vi "Unflatten.vi"(8 "error in (no error)":errorcluster, 11 "Pulse Gen Scan in":refnum<class "Pulse Gen Scan.lvclass">) -> (0 "error out":errorcluster, 3 "Pulse Gen Scan out":refnum<class "Pulse Gen Scan.lvclass">)   [LabVIEW 2009, in "Pulse Gen Scan.lvclass"]
uses:
  Pulse Gen Scan.lvclass
  Scanner/Scanner.lvclass
  Global/File Locations.vi
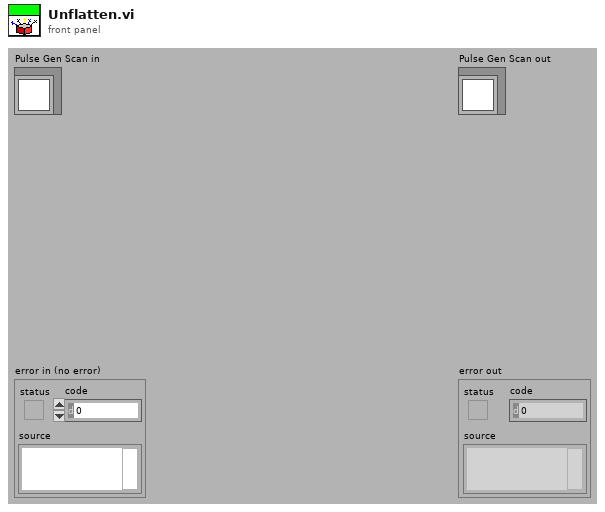
[diagram p1: front panel]
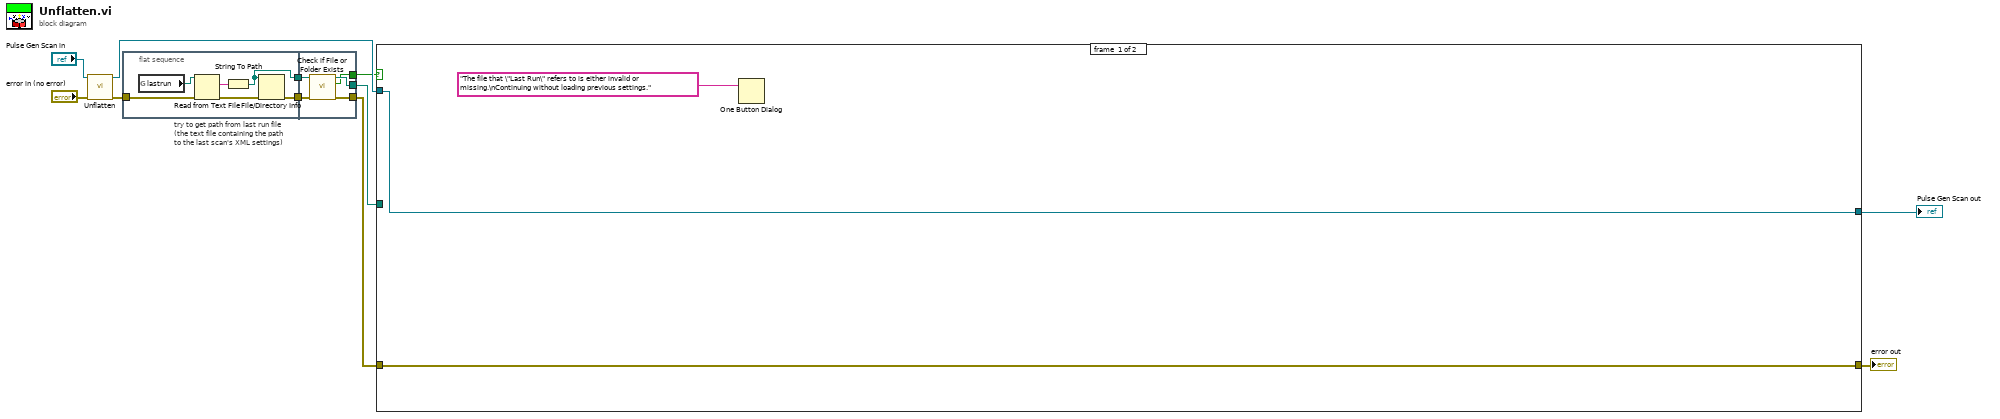
[diagram p0: block diagram]
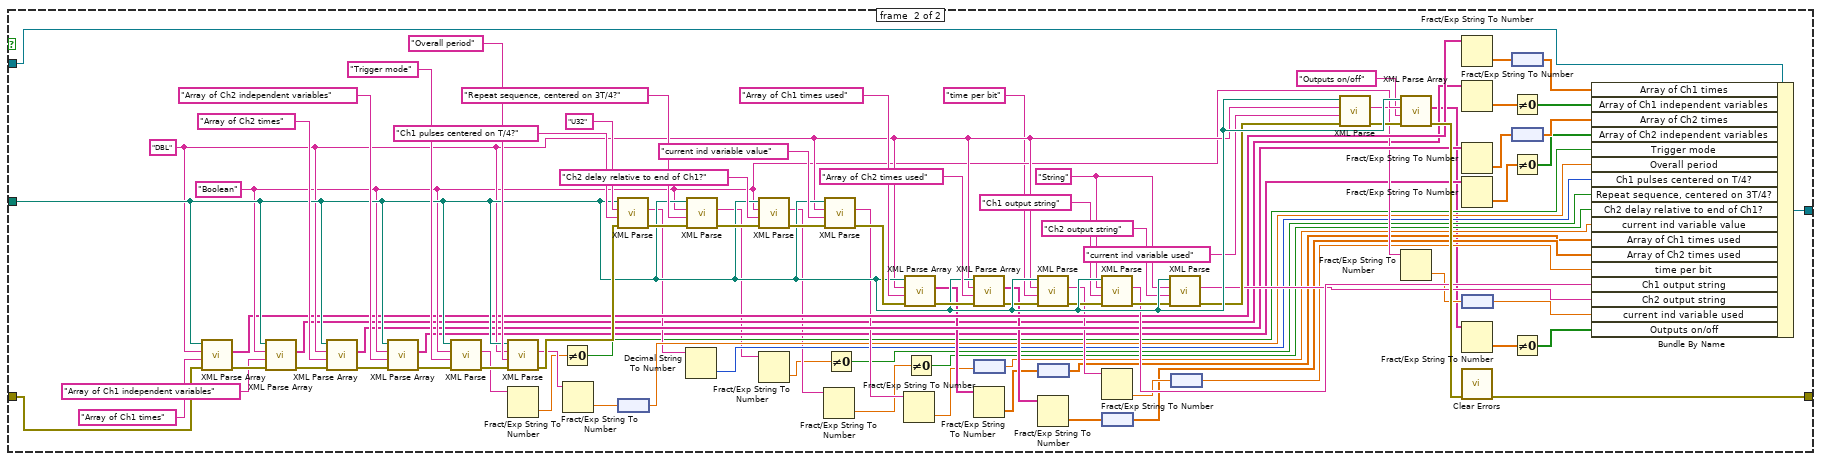
[diagram p2: hidden frame]
diagram:
  n1 = call-parent "Unflatten.vi"("error in (no error)"="error in (no error)", "Scanner in"="Pulse Gen Scan in") -> ("error out"=w7:errorcluster, "Scanner out"=w11:refnum<class "Pulse Gen Scan.lvclass">)  [unwired: 8 in]
  n2 = flat-sequence "try to get path from last run file\n(the text file containing the path\nto the last scan's XML settings)" {
    tunnel: w7 -> [w13]
    tunnel: [w17] -> w3
    tunnel: [w12] -> w2
    tunnel: [w20] -> w6
    tunnel: [w19] -> w5
    tunnel: w3 -> [w22]
    tunnel: w2 -> [w21]
    tunnel: [w18] -> w1
    frame #0 {
      n3 = global read "File Locations.vi" "lastrun"() -> (w15:path)
      n4 = Read from Text File(file (use dialog)=w15, error in=w13) -> (text=w16:string, error out=w14:errorcluster)  [unwired: 4 out]
      n5 = String To Path(string=w16) -> (path=w17:path)
      n6 = File/Directory Info(path=w17, error in=w14) -> (error out=w12:errorcluster)  [unwired: 6 out]
    }
    frame #1 {
      n7 = call <vilib>:"Check if File or Folder Exists.vi"("error in (no error)"=w21, "path"=w22) -> ("error out"=w20:errorcluster, "file or folder exists?"=w18:bool, "dup path"=w19:path)  [unwired: 7 in]
    }
  }
  n8 = case shown="True" w1 {
    tunnel: w11 -> [w24 w114]
    tunnel: [w24 w113] -> w8
    tunnel: w6 -> [w23 w112]
    tunnel: w5 -> [_ w87]
    tunnel: [w23 w26] -> w4
    frame #0 {
      n9 = One Button Dialog(message="The file that \"Last Run\" refers to is either invalid or missing.\nContinuing without loading previous settings.") -> ()  [unwired: 1 in, 1 out]
    }
    frame #1 {
      w86 = "String"
      w84 = "Boolean"
      w85 = "DBL"
      n10 = call "XML Parse Array.vi"("error in (no error)"=w112, "Name String"="Array of Ch1 times", "Type String"=w85, "Path"=w87) -> ("error out"=w111:errorcluster, "Array"=w70:string[])  [unwired: 5 in]
      n11 = call "XML Parse Array.vi"("error in (no error)"=w111, "Name String"="Array of Ch1 independent variables", "Type String"=w84, "Path"=w87) -> ("error out"=w110:errorcluster, "Array"=w44:string[])  [unwired: 5 in]
      n12 = call "XML Parse Array.vi"("error in (no error)"=w110, "Name String"="Array of Ch2 times", "Type String"=w85, "Path"=w87) -> ("error out"=w109:errorcluster, "Array"=w69:string[])  [unwired: 5 in]
      n13 = call "XML Parse Array.vi"("error in (no error)"=w109, "Name String"="Array of Ch2 independent variables", "Type String"=w84, "Path"=w87) -> ("error out"=w104:errorcluster, "Array"=w41:string[])  [unwired: 5 in]
      n14 = call "XML Parse.vi"("error in (no error)"=w104, "Name String"="Trigger mode", "Type String"=w84, "Path"=w87) -> ("error out"=w103:errorcluster, "String Out"=w36:string)  [unwired: 6 in]
      n15 = call "XML Parse.vi"("error in (no error)"=w103, "Name String"="Overall period", "Type String"=w85, "Path"=w87) -> ("error out"=w102:errorcluster, "String Out"=w68:string)  [unwired: 6 in]
      n16 = Fract/Exp String To Number(string=w36) -> (number=w37:dbl)  [unwired: 3 in, 1 out]
      n17 = Not Equal To 0?(x=w37) -> (x != 0?=w38:bool)
      n18 = Fract/Exp String To Number(string=w68) -> (number=w51:dbl)  [unwired: 3 in, 1 out]
      n19 = call "XML Parse.vi"("error in (no error)"=w102, "Name String"="Ch1 pulses centered on T/4?", "Type String"="U32", "Path"=w87) -> ("error out"=w101:errorcluster, "String Out"=w46:string)  [unwired: 6 in]
      n20 = node(w51) -> (w52:dbl[unit])
      n21 = Decimal String To Number(string=w46) -> (number=w45:i32)  [unwired: 2 in, 1 out]
      n22 = call "XML Parse.vi"("error in (no error)"=w101, "Name String"="Repeat sequence, centered on 3T/4?", "Type String"=w84, "Path"=w87) -> ("error out"=w100:errorcluster, "String Out"=w35:string)  [unwired: 6 in]
      n23 = call "XML Parse.vi"("error in (no error)"=w100, "Name String"="Ch2 delay relative to end of Ch1?", "Type String"=w84, "Path"=w87) -> ("error out"=w99:errorcluster, "String Out"=w34:string)  [unwired: 6 in]
      n24 = Fract/Exp String To Number(string=w35) -> (number=w33:dbl)  [unwired: 3 in, 1 out]
      n25 = Fract/Exp String To Number(string=w34) -> (number=w30:dbl)  [unwired: 3 in, 1 out]
      n26 = call "XML Parse.vi"("error in (no error)"=w99, "Name String"="current ind variable value", "Type String"=w85, "Path"=w87) -> ("error out"=w89:errorcluster, "String Out"=w67:string)  [unwired: 6 in]
      n27 = Not Equal To 0?(x=w33) -> (x != 0?=w32:bool)
      n28 = Fract/Exp String To Number(string=w67) -> (number=w53:dbl)  [unwired: 3 in, 1 out]
      n29 = call "XML Parse Array.vi"("error in (no error)"=w89, "Name String"="Array of Ch1 times used", "Type String"=w85, "Path"=w87) -> ("error out"=w88:errorcluster, "Array"=w66:string[])  [unwired: 5 in]
      n30 = Not Equal To 0?(x=w30) -> (x != 0?=w31:bool)
      n31 = call "XML Parse Array.vi"("error in (no error)"=w88, "Name String"="Array of Ch2 times used", "Type String"=w85, "Path"=w87) -> ("error out"=w83:errorcluster, "Array"=w65:string[])  [unwired: 5 in]
      n32 = node(w53) -> (w54:dbl[unit])
      n33 = Fract/Exp String To Number(string=w66) -> (number=w56:dbl[])  [unwired: 3 in, 1 out]
      n34 = call "XML Parse.vi"("error in (no error)"=w83, "Name String"="time per bit", "Type String"=w85, "Path"=w87) -> ("error out"=w82:errorcluster, "String Out"=w64:string)  [unwired: 6 in]
      n35 = node(w56) -> (w55:dbl[unit][])
      n36 = Fract/Exp String To Number(string=w65) -> (number=w57:dbl[])  [unwired: 3 in, 1 out]
      n37 = call "XML Parse.vi"("error in (no error)"=w82, "Name String"="Ch1 output string", "Type String"=w86, "Path"=w87) -> ("error out"=w81:errorcluster, "String Out"=w72:string)  [unwired: 6 in]
      n38 = Fract/Exp String To Number(string=w64) -> (number=w60:dbl)  [unwired: 3 in, 1 out]
      n39 = node(w57) -> (w58:dbl[unit][])
      n40 = call "XML Parse.vi"("error in (no error)"=w81, "Name String"="Ch2 output string", "Type String"=w86, "Path"=w87) -> ("error out"=w80:errorcluster, "String Out"=w71:string)  [unwired: 6 in]
      n41 = node(w60) -> (w59:dbl[unit])
      n42 = call "XML Parse.vi"("error in (no error)"=w80, "Name String"="current ind variable used", "Type String"=w85, "Path"=w87) -> ("error out"=w79:errorcluster, "String Out"=w63:string)  [unwired: 6 in]
      n43 = call "XML Parse Array.vi"("error in (no error)"=w79, "Name String"="Outputs on/off", "Type String"=w84, "Path"=w87) -> ("error out"=w78:errorcluster, "Array"=w27:string[])  [unwired: 5 in]
      n44 = Fract/Exp String To Number(string=w63) -> (number=w61:dbl)  [unwired: 3 in, 1 out]
      n45 = Fract/Exp String To Number(string=w70) -> (number=w47:dbl[])  [unwired: 3 in, 1 out]
      n46 = Fract/Exp String To Number(string=w44) -> (number=w43:dbl[])  [unwired: 3 in, 1 out]
      n47 = Fract/Exp String To Number(string=w69) -> (number=w50:dbl[])  [unwired: 3 in, 1 out]
      n48 = Fract/Exp String To Number(string=w41) -> (number=w40:dbl[])  [unwired: 3 in, 1 out]
      n49 = node(w61) -> (w62:dbl[unit])
      n50 = Fract/Exp String To Number(string=w27) -> (number=w28:dbl[])  [unwired: 3 in, 1 out]
      n51 = call <vilib>:"Clear Errors.vi"("error in (no error)"=w78) -> ("error out"=w26:errorcluster)  [unwired: 6 in]
      n52 = node(w47) -> (w48:dbl[unit][])
      n53 = Not Equal To 0?(x=w43) -> (x != 0?=w42:bool[])
      n54 = node(w50) -> (w49:dbl[unit][])
      n55 = Not Equal To 0?(x=w40) -> (x != 0?=w39:bool[])
      n56 = Not Equal To 0?(x=w28) -> (x != 0?=w29:bool[])
      n57 = Bundle By Name(cluster=w114, "Array of Ch1 times"=w48, "Array of Ch1 independent variables"=w42, "Array of Ch2 times"=w49, "Array of Ch2 independent variables"=w39, "Trigger mode"=w38, "Overall period"=w52, "Ch1 pulses centered on T/4?"=w45, "Repeat sequence, centered on 3T/4?"=w32, "Ch2 delay relative to end of Ch1?"=w31, "current ind variable value"=w54, "Array of Ch1 times used"=w55, "Array of Ch2 times used"=w58, "time per bit"=w59, "Ch1 output string"=w72, "Ch2 output string"=w71, "current ind variable used"=w62, "Outputs on/off"=w29) -> (w113:refnum<class "Pulse Gen Scan.lvclass">)
    }
  }
  "error out" <- w4
  "Pulse Gen Scan out" <- w8
